vi "FindLocalizedString.vi"(9 "LangIndex":u32, 10 "LocalizationFileContent":T1, 11 "WordIndex":u32) -> (2 "Found":bool, 3 "LocalizedString":string)   [LabVIEW 2012]
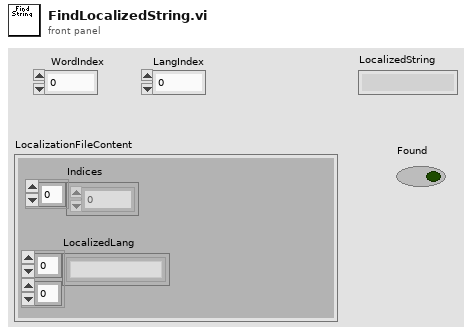
[diagram p1: front panel]
types:
  T1 = cluster{"Indices":u32[], "LocalizedLang":string[][]}
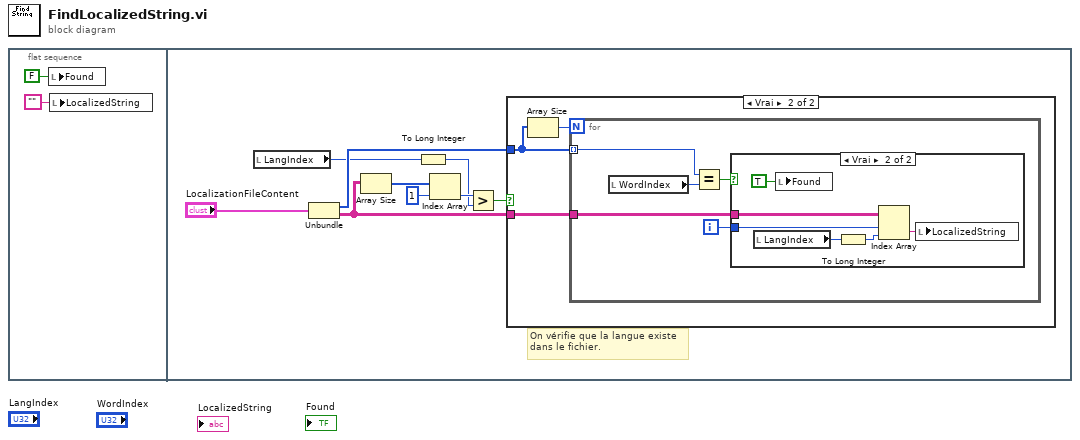
[diagram p0: block diagram]
diagram:
  n1 = flat-sequence {
    frame #0 {
      n2 = local write "Found"(FALSE) -> ()
      n3 = local write "LocalizedString"("") -> ()
    }
    frame #1 {
      # "On vérifie que la langue existe\ndans le fichier."
      n4 = local read "LangIndex"() -> (w4:u32)
      n5 = Unbundle("LocalizationFileContent") -> ("Indices"=w10:u32[], "LocalizedLang"=w5:string[][])
      n6 = Array Size(array=w5) -> (size(s)=w8:i32[])
      n7 = To Long Integer(number=w4) -> (32bit integer=w3:i32)
      n8 = Index Array(array=w8, index=1) -> (element=w6:i32)
      n9 = Greater?(x=w6, y=w3) -> (0:w9:bool)
      n10 = case shown="Vrai" w9 {
        tunnel: w10 -> [_ w13]
        tunnel: w5 -> [_ w12]
        frame False {
        }
        frame True {
          n11 = Array Size(array=w13) -> (size(s)=w14:i32)
          n12 = for {
            N: w14 -> [_]
            tunnel: w13 -> [w18] mode=indexing
            tunnel: w12 -> [w17]
            i -> [w15]
            n13 = local read "WordIndex"() -> (w16:u32)
            n14 = Equal?(x=w18, y=w16) -> (x = y?=w19:bool)
            n15 = case shown="Vrai" w19 {
              tunnel: w17 -> [_ w23]
              tunnel: w15 -> [_ w22]
              frame False {
              }
              frame True {
                n16 = local read "LangIndex"() -> (w21:u32)
                n17 = local write "Found"(TRUE) -> ()
                n18 = To Long Integer(number=w21) -> (32bit integer=w20:i32)
                n19 = Index Array(array=w23, index (row)=w22, index (col)=w20) -> (element=w24:string)
                n20 = local write "LocalizedString"(w24) -> ()
              }
            }
          }
        }
      }
    }
  }
